vi "h5_init_2D.vi"(0 "files":path[](array[path]), 1 "var 0":string, 2 "v0_config":T1={"hardware"=enum."wait (s)", "options"="", "repeats"=1, "loops"=1, "VISA"="", "override_VISA"=FALSE} {"loops" min=1; "repeats" min=1}, 3 "v0_num":i32, 5 "RID":string, 11 "error in (no error)":errorcluster, 12 "var 1":string, 13 "v1_config":T1={"hardware"=enum."wait (s)", "options"="", "repeats"=1, "loops"=1, "VISA"="", "override_VISA"=FALSE} {"loops" min=1; "repeats" min=1}, 14 "v1_num":i32) -> (15 "error out":errorcluster)   [LabVIEW 2017, in "tools.lvlib"]
uses:
  tools.lvlib
  core/var_config.ctl
  ctrl/var_list.ctl
  <vilib>/UPVI/lvhdf5/file.llb/LVH5F Operation.ctl
  <vilib>/UPVI/lvhdf5/attribute.llb/Simple H5Awrite (Variant).vi
  <vilib>/UPVI/lvhdf5/attribute.llb/LVH5A Operation.ctl
  <vilib>/UPVI/lvhdf5/attribute.llb/Simple H5Awrite.xnode
  <vilib>/UPVI/lvhdf5/library.llb/HDF5 Ref.ctl
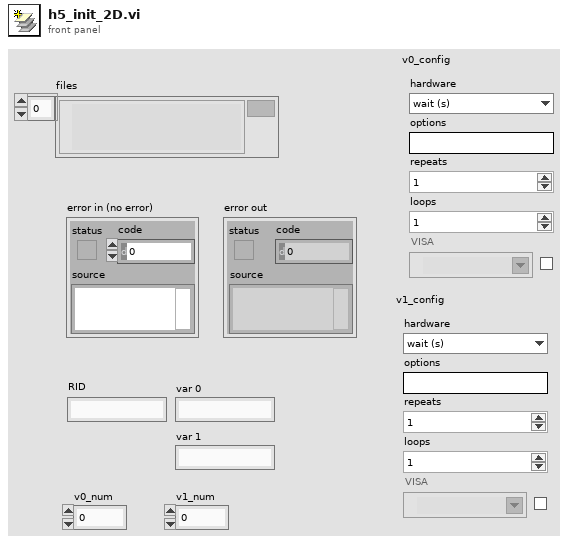
[diagram p1: front panel]
types:
  T1 = typedef "tools.lvlib/var_config.ctl" = cluster{"hardware":T2, "options":string, "repeats":i32, "loops":i32, "VISA":refnum<visa-resource-name>, "override_VISA":bool}
  T2 = typedef "var_list.ctl" = enum16{"none", "AO voltage (V)", "delay (s)", "generic", "microwaves (GHz)", "radiant (nm)", "radiant thg (nm)", "sirah (nm)", "sirah_shg (nm)", "tenma voltage (V)", "wait (s)", "wf_freq (Hz)", "wf_amp (V)", "wf_amp_multi (V)", "wf_offset (V)", "wf_low_level (V)", "wf_high_level (V)", "wf_period (s)", "wf_pulse_width (s)", "wf_sample_rate (Sa/s)", "wf_multi_amp", "wf_multi_freq", "wf_arb_4chan", "WS7 setpoint (nm)"}
  T3 = typedef "Semaphore RefNum" = refnum<k1>
  T4 = typedef "LVH5F Operation.ctl" = enum16{"open", "open or create", "create or replace", "create or replace (with confirmation)", "create", "open (read only)"}
  T5 = typedef "HDF5 Ref.ctl" = refnum<k1>
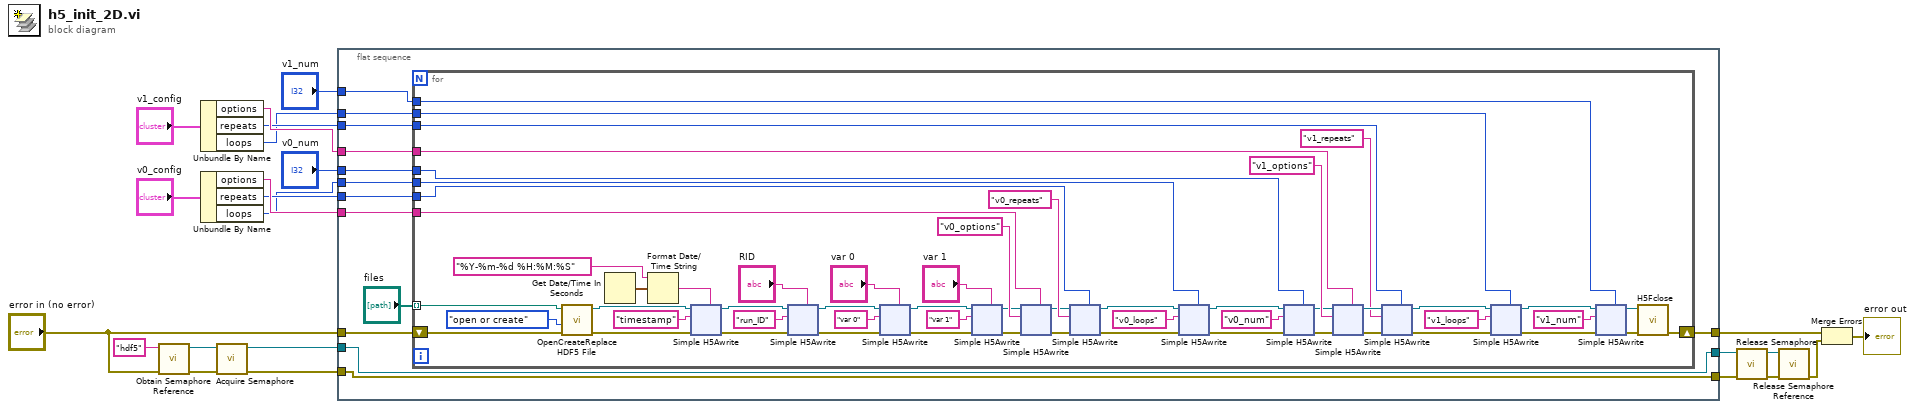
[diagram p0: block diagram]
diagram:
  n1 = call <vilib>:"Obtain Semaphore Reference.vi"("error in (no error)"="error in (no error)", "name (unnamed)"="hdf5") -> ("error out"=w22:errorcluster, "semaphore"=w23:T3)  [unwired: 3 in, 1 out]
  n2 = Unbundle By Name("v1_config") -> ("options"=w7:string, "repeats"=w4:i32, "loops"=w3:i32)
  n3 = Unbundle By Name("v0_config") -> ("options"=w9:string, "repeats"=w6:i32, "loops"=w5:i32)
  n4 = call <vilib>:"Acquire Semaphore.vi"("error in (no error)"=w22, "semaphore"=w23) -> ("error out"=w17:errorcluster, "semaphore out"=w16:T3)  [unwired: 3 in, 1 out]
  n5 = flat-sequence {
    tunnel: "error in (no error)" -> [w33]
    tunnel: w17 -> [w36]
    tunnel: w16 -> [w35]
    tunnel: [w36] -> w15
    tunnel: [w35] -> w14
    tunnel: [w34] -> w13
    tunnel: w9 -> [w31]
    tunnel: w7 -> [w30]
    tunnel: w6 -> [w29]
    tunnel: w5 -> [w28]
    tunnel: w4 -> [w27]
    tunnel: w3 -> [w26]
    tunnel: "v1_num" -> [w25]
    tunnel: "v0_num" -> [w24]
    frame #0 {
      n6 = for {
        shift-right: [w76] -> w34
        shift-left: w33 -> [w75]
        tunnel: "files" -> [w74] mode=indexing
        tunnel: w31 -> [w67]
        tunnel: w30 -> [w55]
        tunnel: w29 -> [w63]
        tunnel: w28 -> [w62]
        tunnel: w27 -> [w50]
        tunnel: w26 -> [w49]
        tunnel: w25 -> [w45]
        tunnel: w24 -> [w44]
        n7 = call <vilib>:"OpenCreateReplace HDF5 File.vi"("error in (no error)"=w75, "function (open or create)"=LVH5F_Operation."open or create", "path"=w74) -> ("error out"=w91:errorcluster, "HDF5 Ref out"=w92:T5)  [unwired: 5 in]
        n8 = Get Date/Time In Seconds() -> (seconds since 1Jan1904=w88:timestamp)
        n9 = Format Date/Time String(time format string (%c)="%Y-%m-%d %H:%M:%S", seconds (now)=w88) -> (date/time string=w87:string)  [unwired: 1 in]
        n10 = xnode "Simple H5Awrite"("HDF5 Ref"=w92, "Name"="timestamp", "error in (no error)"=w91, "Value"=w87) -> ("HDF5 Ref out"=w85:T5, "error out"=w82:errorcluster)  [unwired: 1 in]
        n11 = xnode "Simple H5Awrite"("HDF5 Ref"=w85, "Name"="run_ID", "error in (no error)"=w82, "Value"="RID") -> ("HDF5 Ref out"=w84:T5, "error out"=w83:errorcluster)  [unwired: 1 in]
        n12 = xnode "Simple H5Awrite"("HDF5 Ref"=w84, "Name"="var 0", "error in (no error)"=w83, "Value"="var 0") -> ("HDF5 Ref out"=w72:T5, "error out"=w73:errorcluster)  [unwired: 1 in]
        n13 = xnode "Simple H5Awrite"("HDF5 Ref"=w72, "Name"="var 1", "error in (no error)"=w73, "Value"="var 1") -> ("HDF5 Ref out"=w71:T5, "error out"=w70:errorcluster)  [unwired: 1 in]
        n14 = xnode "Simple H5Awrite"("HDF5 Ref"=w71, "Name"="v0_options", "error in (no error)"=w70, "Value"=w67) -> ("HDF5 Ref out"=w65:T5, "error out"=w64:errorcluster)  [unwired: 1 in]
        n15 = xnode "Simple H5Awrite"("HDF5 Ref"=w65, "Name"="v0_repeats", "error in (no error)"=w64, "Value"=w63) -> ("HDF5 Ref out"=w60:T5, "error out"=w61:errorcluster)  [unwired: 1 in]
        n16 = xnode "Simple H5Awrite"("HDF5 Ref"=w60, "Name"="v0_loops", "error in (no error)"=w61, "Value"=w62) -> ("HDF5 Ref out"=w41:T5, "error out"=w42:errorcluster)  [unwired: 1 in]
        n17 = xnode "Simple H5Awrite"("HDF5 Ref"=w41, "Name"="v0_num", "error in (no error)"=w42, "Value"=w44) -> ("HDF5 Ref out"=w39:T5, "error out"=w40:errorcluster)  [unwired: 1 in]
        n18 = xnode "Simple H5Awrite"("HDF5 Ref"=w39, "Name"="v1_options", "error in (no error)"=w40, "Value"=w55) -> ("HDF5 Ref out"=w57:T5, "error out"=w58:errorcluster)  [unwired: 1 in]
        n19 = xnode "Simple H5Awrite"("HDF5 Ref"=w57, "Name"="v1_repeats", "error in (no error)"=w58, "Value"=w50) -> ("HDF5 Ref out"=w51:T5, "error out"=w52:errorcluster)  [unwired: 1 in]
        n20 = xnode "Simple H5Awrite"("HDF5 Ref"=w51, "Name"="v1_loops", "error in (no error)"=w52, "Value"=w49) -> ("HDF5 Ref out"=w38:T5, "error out"=w37:errorcluster)  [unwired: 1 in]
        n21 = xnode "Simple H5Awrite"("HDF5 Ref"=w38, "Name"="v1_num" ("v1_num"), "error in (no error)"=w37, "Value"=w45) -> ("HDF5 Ref out"=w43:T5, "error out"=w46:errorcluster)  [unwired: 1 in]
        n22 = call <vilib>:"H5Fclose.vi"("error in (no error)"=w46, "HDF5 Ref"=w43) -> ("error out"=w76:errorcluster)  [unwired: 7 in]
      }
    }
  }
  n23 = call <vilib>:"Release Semaphore.vi"("error in (no error)"=w15, "semaphore"=w14) -> ("error out"=w20:errorcluster, "semaphore out"=w19:T3)  [unwired: 4 in]
  n24 = call <vilib>:"Release Semaphore Reference.vi"("error in (no error)"=w20, "semaphore"=w19) -> ("error out"=w12:errorcluster)  [unwired: 8 in, 1 out]
  n25 = Merge Errors(w13, w12) -> (→"error out":errorcluster)
